vi "VI Server_TREE_Clear.vi"(7 "Label":string, 8 "error in":errorcluster, 9 "Tree.Ref":refnum<vi>, 11 "VI Server.RefsCluster":T1) -> (0 "error out":errorcluster, 1 "Tree.Ref.DUP":refnum<vi>, 3 "VI Server.RefsCluster.DUP":T1)   [LabVIEW 2020]
uses:
  VI Server_TypeDefs/VI Server_RefsCluster.ctl
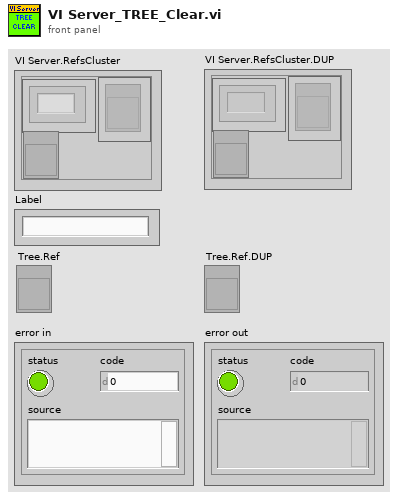
[diagram p1: front panel]
types:
  T1 = typedef "VI Server_RefsCluster.ctl" = cluster{"Labels":string[], "Refs":refnum<vi>[], "VI Ref":refnum<vi>}
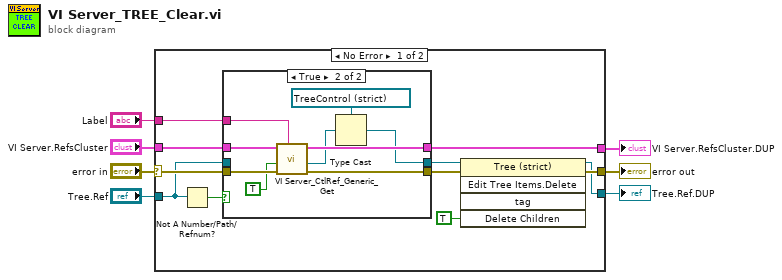
[diagram p0: block diagram]
diagram:
  n1 = case shown="No Error" "error in" {
    selector: "error in" -> [w18 w32]
    tunnel: [w10 w32] -> w6
    tunnel: "VI Server.RefsCluster" -> [w17 w31]
    tunnel: [w16 w31] -> w4
    tunnel: "Label" -> [w15 _]
    tunnel: "Tree.Ref" -> [w13 _]
    tunnel: [w8 _] -> w2
    frame No Error {
      n2 = Not A Number/Path/Refnum?(number/path/refnum=w13) -> (NaN/Path/Refnum?=w14:bool)
      n3 = case shown="True" w14 {
        tunnel: w18 -> [w21 w30]
        tunnel: w17 -> [w19 w29]
        tunnel: [w19 w28] -> w16
        tunnel: w15 -> [_ w27]
        tunnel: [w20 w25] -> w9
        tunnel: [w21 w24] -> w11
        tunnel: w13 -> [w20 _]
        frame False {
        }
        frame True {
          n4 = call "VI Server_CtlRef_Generic_Get.vi"("Control.Label"=w27, "error in"=w30, "SingleInstance"=TRUE, "VI Server.RefsCluster"=w29) -> ("error out"=w24:errorcluster, "Control.Ref.Generic"=w26:refnum<vi>, "VI Server.RefsCluster.DUP"=w28:T1)  [unwired: 5 in]
          n5 = Type Cast(type=refnum<vi> refnum ("Test.Tree"), x=w26) -> (*(type *) &x=w25:refnum<vi>)
        }
      }
      n6 = invoke on="Invoke Node" class="Tree (strict)" method="Edit Tree Items.Delete"(reference=w9, error in=w11, "Delete Children"=TRUE ("Delete Children?")) -> (reference out=w8:refnum<vi>, error out=w10:errorcluster)  [unwired: 2 in, 3 out]
    }
    frame Error {
    }
  }
  "VI Server.RefsCluster.DUP" <- w4
  "error out" <- w6
  "Tree.Ref.DUP" <- w2
